vi "capt_scaling.vi"(8 "error in":errorcluster, 10 "Gain":sgl format="%.6e", 11 "Offset":sgl format="%.6e") -> (0 "error out":errorcluster)   [LabVIEW 2013]
uses:
  GlobalVariables/CaptParameters.vi
panel:
  in  "Address":u8=250 format="%x"
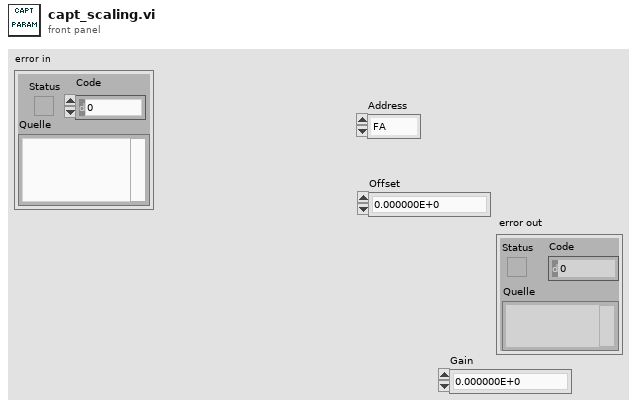
[diagram p1: front panel]
types:
  T1 = cluster{"baudrate":u32, "databits":u16, "paritybit":u16, "stopbits":u16, "flux control":u16, "Port":string, "Register Address":u16, "Serial Parameters":cluster{"Mode":enum16{"RTU", "ASCII"}, "Slave Address":u8}, "Timeout":u32}
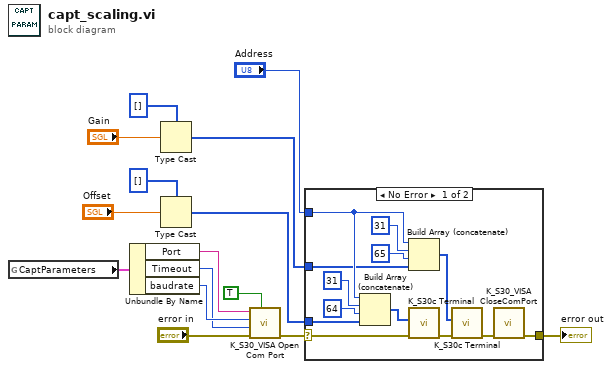
[diagram p0: block diagram]
diagram:
  n1 = global read "CaptParameters.vi" "CaptParameters"() -> (w14:T1)
  n2 = Unbundle By Name(w14) -> ("Port"=w13:string, "Timeout"=w10:u32, "baudrate"=w12:u32)
  n3 = Type Cast(type=u8[] [] ("response"), x="Gain") -> (*(type *) &x=w1:u8[])
  n4 = Type Cast(type=u8[] [] ("response"), x="Offset") -> (*(type *) &x=w5:u8[])
  n5 = call "K_S30_VISA Open Com Port.vi"("RS-converter:\necho"=TRUE ("RS-converter: echo"), "error in (no error)"="error in", "timeout"=w10, "Baudrate"=w12, "VISA resource name"=w13) -> ("error out"=w4:errorcluster)  [unwired: 3 in, 1 out]
  n6 = case shown="No Error" w4 {
    selector: w4 -> [w26 w29]
    tunnel: "Address" -> [w21 _]
    tunnel: [w17 w29] -> w8
    tunnel: w5 -> [w25 _]
    tunnel: w1 -> [w18 _]
    frame No Error {
      n7 = Build Array (concatenate)(w21, u8 31 ("Element"), u8 64 ("Register"), w25) -> (w27:u8[])
      n8 = Build Array (concatenate)(w21, u8 31 ("Element"), u8 65 ("Register"), w18) -> (w22:u8[])
      n9 = call "K_S30c Terminal.vi"("error in"=w26, "request"=w27) -> ("error out"=w24:errorcluster)  [unwired: 4 in, 1 out]
      n10 = call "K_S30c Terminal.vi"("error in"=w24, "request"=w22) -> ("error out"=w16:errorcluster)  [unwired: 4 in, 1 out]
      n11 = call "K_S30_VISA CloseComPort.vi"("error in (not connected)"=w16) -> ("Fehlerausgang"=w17:errorcluster)  [unwired: 6 in]
    }
    frame Error {
    }
  }
  "error out" <- w8
